vi "Send_Voltage.vi"(1 "error in":errorcluster, 2 "Voltage":dbl) -> (0 "error out":errorcluster)   [LabVIEW 2010]
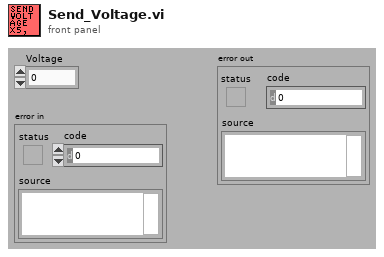
[diagram p1: front panel]
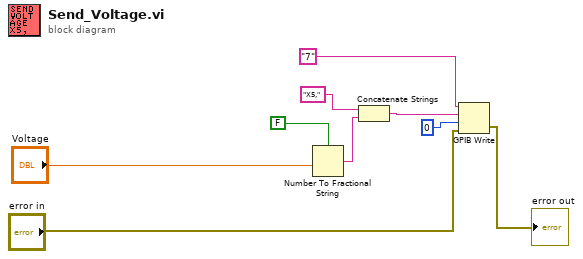
[diagram p0: block diagram]
diagram:
  n1 = Number To Fractional String(use system decimal point (T)=FALSE, number="Voltage") -> (F-format string=w4:string)  [unwired: 2 in]
  n2 = Concatenate Strings("X5,", w4) -> (w6:string)
  n3 = GPIB Write(0:"7", 1:w6, 2:0, 3:"error in") -> (6:→"error out":errorcluster)  [unwired: 1 in, 1 out]
